vi "VI Tree.vi"   [LabVIEW 2023, in "Longer Pump dLSP501 Series.lvlib"]
doc: "This is the instrument driver for the <INSTRUMENT NAME>. The VI Tree displays all the user-callable VIs of the instrument driver in an organized table."
uses:
  <instrlib>/Longer Pump dLSP501 Modbus RTU Series/Longer Pump dLSP501 Series.lvlib
  <instrlib>/Longer Pump dLSP501 Modbus RTU Series/Private/Initialize - Individual Address.vi
panel:
  # "(c) 2025 Longer Precision Pump Co. Ltd.  ALL RIGHTS RESERVED."
  # "SEE DIAGRAM\nFOR VI TREE."
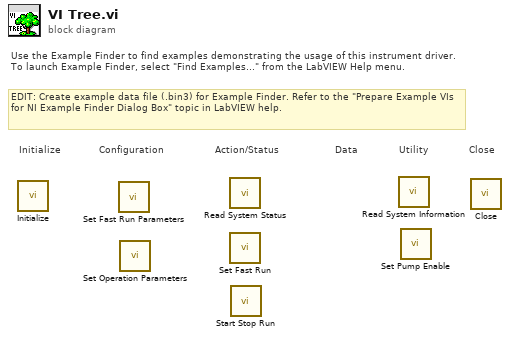
[diagram p0: block diagram]
diagram:
  # "EDIT: Create example data file (.bin3) for Example Finder. Refer to the \"Prepare Example VIs for NI Example Finder Dialog Box\" topic in LabVIEW help."
  # "Use the Example Finder to find examples demonstrating the usage of this instrument driver.\nTo launch Example Finder, select \"Find Examples...\" from the LabVIEW Help menu."
  # "Configuration"
  # "Utility"
  # "Data"
  # "Action/Status"
  # "Close"
  # "Initialize"
  n1 = call-poly <instrlib>:"Initialize.vi"() -> ()  [unwired: 8 in, 3 out]
  n2 = call <instrlib>:"Set Fast Run Parameters.vi"() -> ()  [unwired: 10 in, 2 out]
  n3 = call <instrlib>:"Set Operation Parameters.vi"() -> ()  [unwired: 10 in, 2 out]
  n4 = call <instrlib>:"Read System Status.vi"() -> ()  [unwired: 8 in, 4 out]
  n5 = call <instrlib>:"Set Fast Run.vi"() -> ()  [unwired: 10 in, 2 out]
  n6 = call <instrlib>:"Start Stop Run.vi"() -> ()  [unwired: 10 in, 2 out]
  n7 = call <instrlib>:"Read System Information.vi"() -> ()  [unwired: 6 in, 6 out]
  n8 = call <instrlib>:"Set Pump Enable.vi"() -> ()  [unwired: 10 in, 2 out]
  n9 = call <instrlib>:"Close.vi"() -> ()  [unwired: 11 in, 1 out]
